vi "Stop FFMpeg Process.vi"(8 "error in (no error)":errorcluster, 11 "FFMpegProcess":T1) -> (0 "error out":errorcluster)   [LabVIEW 2024]
doc: "Use this template to build a VI to use as a subVI."
uses:
  controls/FFMpegRef.ctl
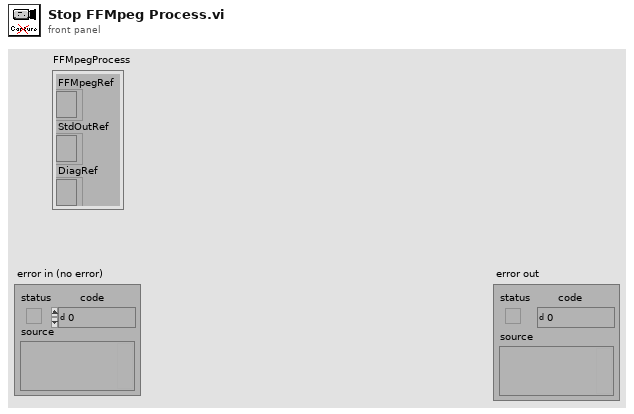
[diagram p1: front panel]
types:
  T1 = typedef "FFMpegRef.ctl" = cluster{"FFMpegRef":refnum<k24>, "StdOutRef":refnum<k24>, "DiagRef":refnum<k24>}
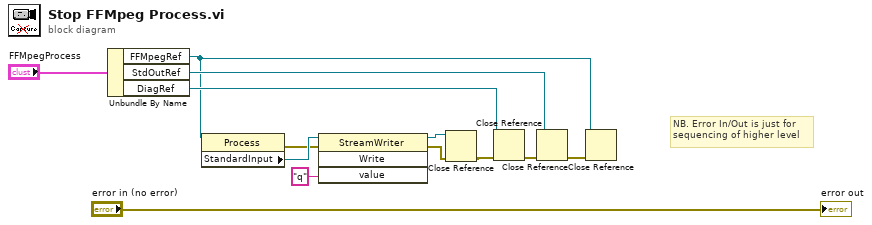
[diagram p0: block diagram]
diagram:
  # "NB. Error In/Out is just for \nsequencing of higher level"
  n1 = Unbundle By Name("FFMpegProcess") -> ("FFMpegRef"=w2:refnum<k24>, "StdOutRef"=w9:refnum<k24>, "DiagRef"=w10:refnum<k24>)
  n2 = property class="Process"(reference=w2) -> (error out=w6:errorcluster, "StandardInput"=w7:refnum<k24>)  [unwired: 1 in, 1 out]
  n3 = invoke class="StreamWriter" method="Write"(reference=w7, error in=w6, "value"="q") -> (reference out=w3:refnum<k24>, error out=w5:errorcluster)  [unwired: 1 in, 2 out]
  n4 = Close Reference(reference=w3, error in (no error)=w5) -> (error out=w4:errorcluster)
  n5 = Close Reference(reference=w10, error in (no error)=w4) -> (error out=w12:errorcluster)
  n6 = Close Reference(reference=w9, error in (no error)=w12) -> (error out=w11:errorcluster)
  n7 = Close Reference(reference=w2, error in (no error)=w11) -> ()  [unwired: 1 out]
  "error out" <- "error in (no error)"
